vi "sectortemp.vi"() -> ()   [LabVIEW 2022 SP3]
uses:
  <vilib>/Utility/file.llb/Write To Spreadsheet File (DBL).vi
panel:
  in  "z 2":dbl[][](array[numeric])=array250x318[79500 elements] format="%.2f"
  in  "y 2":dbl[][](array[numeric]) format="%.2f"
  in  "x 2":dbl[][](array[numeric]) format="%.2f"
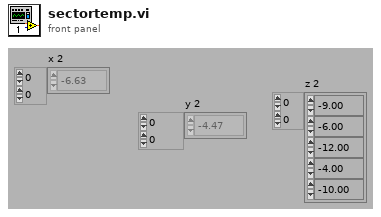
[diagram p1: front panel]
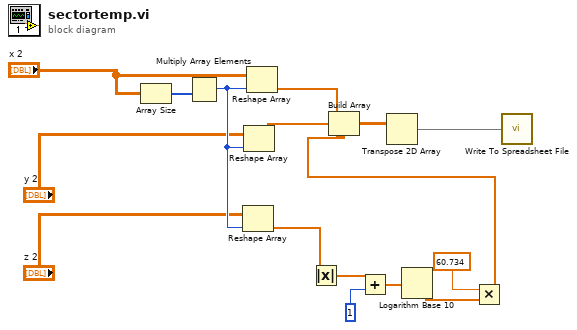
[diagram p0: block diagram]
diagram:
  n1 = Array Size(array="x 2") -> (size(s)=w16:i32[])
  n2 = Multiply Array Elements(1:w16) -> (0:w15:i32)
  n3 = Reshape Array("z 2", w15) -> (w6:dbl[])
  n4 = Reshape Array("y 2", w15) -> (w13:dbl[])
  n5 = Reshape Array("x 2", w15) -> (w14:dbl[])
  n6 = Absolute Value(x=w6) -> (abs(x)=w1:dbl[])
  n7 = Add(x=w1, y=1) -> (x+y=w8:dbl[])
  n8 = Logarithm Base 10(1:w8) -> (0:w10:dbl[])
  n9 = Multiply(x=60.734, y=w10) -> (x*y=w7:dbl[])
  n10 = Build Array(w14, w13, w7) -> (w12:dbl[][])
  n11 = Transpose 2D Array(2D array=w12) -> (transposed array=w11:dbl[][])
  n12 = call-poly <vilib>:"Write To Spreadsheet File.vi"("2D data"=w11) -> ()  [unwired: 5 in, 3 out]
